vi "Find Center - Copy.vi"(7 "Tray Number":dbl format="%#_13g", 9 "XYZTheta":dbl[](array[numeric]), 11 "Gantry In":refnum<k24>) -> (1 "XYZTheta Centers":dbl[][](array[numeric]), 3 "Gantry Out":refnum<k24>)   [LabVIEW 2019, in "Assembly Tray.lvclass"]
uses:
  Assembly Tray.lvclass
  Find Tray.ctl
  Controller/Camera/Machine Vision.ctl
  C:/Program Files (x86)/Aerotech/A3200/LabVIEW/2010/Bin/Aerotech.A3200.dll
  Program Files (x86)/Aerotech/A3200/LabVIEW/2010/Bin/Aerotech.A3200.dll
  Controller/Camera/Camera.lvclass
  Controller/Motion/A3200/A3200.lvclass
panel:
  in  "BCG Values":T1={"Brightness"=128.0, "Contrast"=45.0, "Gamma"=1.0}
  in  "Machine Vision":T2=enum."Tray Fiducials"
  out "Right Fiducial":dbl[](array[numeric])
  out "Left Fiducial":dbl[](array[numeric])
  out "Gantry":dbl[](array[numeric])
  out "Sum":dbl[](array[numeric])
  out "Camera":dbl[](array[numeric])
  in  "Carrier Tray":T3
  out "Image":T4(plugin-control)
  out "Center":dbl[](array[numeric])
  in  "Position Number":i16
  in  "Go to Center":bool
  in  "Calculate":bool
  in  "Record Bottom":bool
  in  "Record Top":bool
  in  "Go to Bottom Fiducial":bool
  in  "Go to Top Fiducial":bool
  in  "Joystick":bool
  in  "Stop":bool
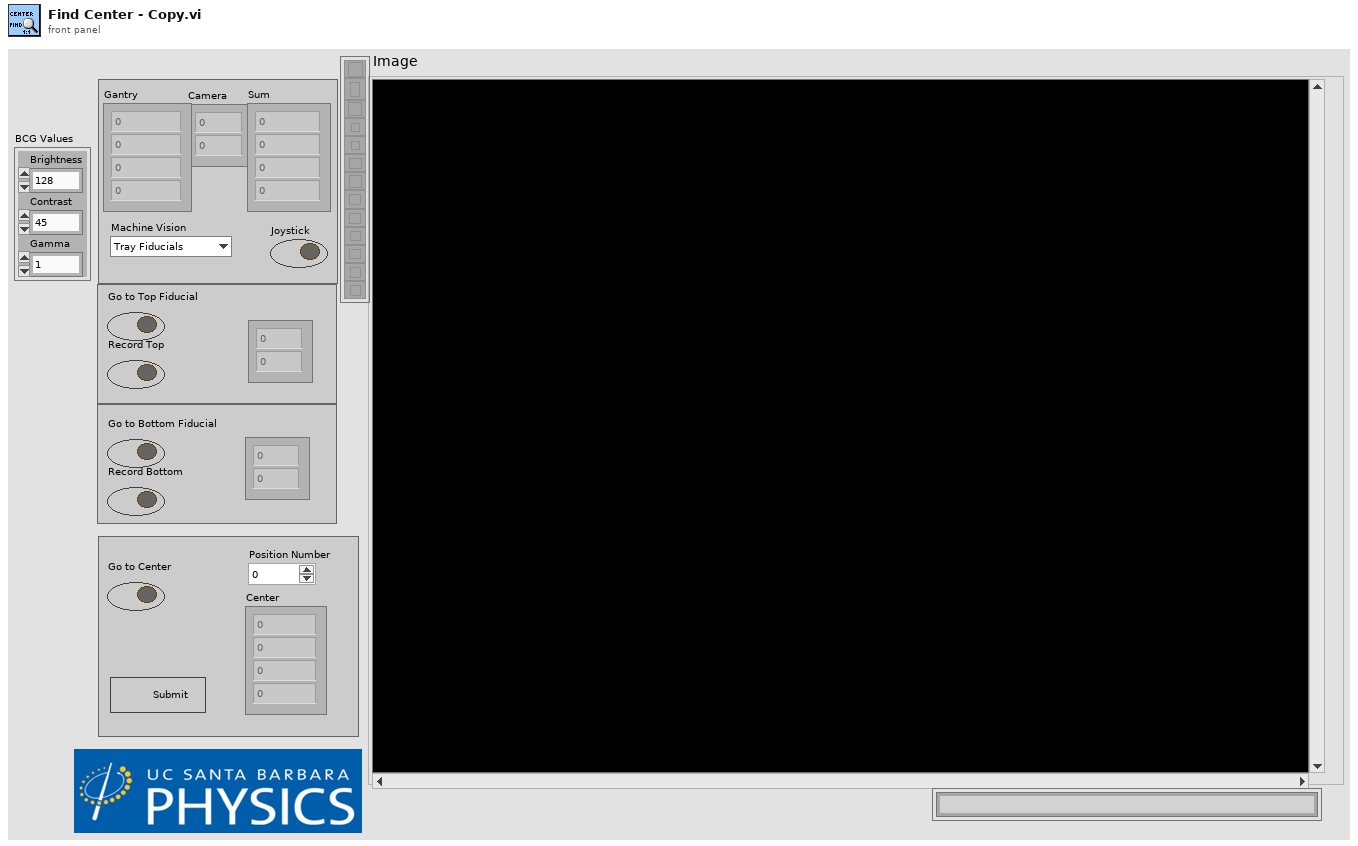
[diagram p1: front panel]
types:
  T1 = cluster{"Brightness":sgl, "Contrast":sgl, "Gamma":sgl}
  T2 = typedef "Camera.lvclass/Machine Vision.ctl" = enum16{"None", "Tray Fiducials", "HPK Silicon", "Hexaboard", "Corner (TL, BR)", "Corner (BL, TR)", "sensor TL", "sensor BL", "sensor TR", "sensor BR", "hexaboard TL", "hexaboard BL", "hexaboard TR", "hexaboard BR"}
  T3 = typedef "Assembly Tray.lvclass/Find Tray.ctl" = cluster{"Gantry Fiducials":dbl[], "Relative Coordinates":dbl[][], "Camera Fiducials":dbl[][], "XYZTheta Centers":dbl[][], "Workspace Center":dbl[], "Syringe Relative Coordinates":dbl[], "Gantry Region":dbl, "Fiducials Path":path, "New Fiducials":dbl[][], "Past Fiducials":dbl[][], "XYZTheta":dbl[], "Position":i32}
  T4 = typedef "IMAQ Image.ctl" = refnum<image>
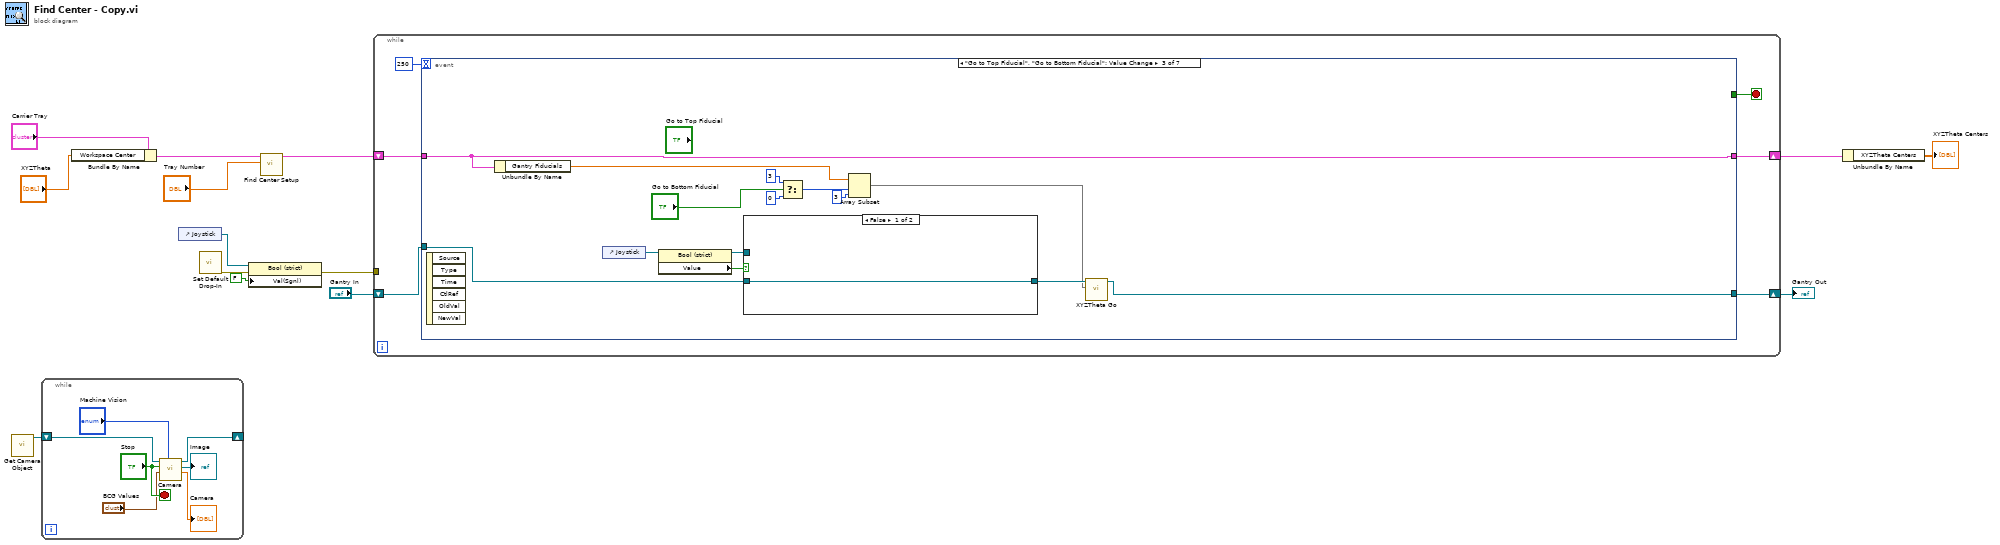
[diagram p0: block diagram]
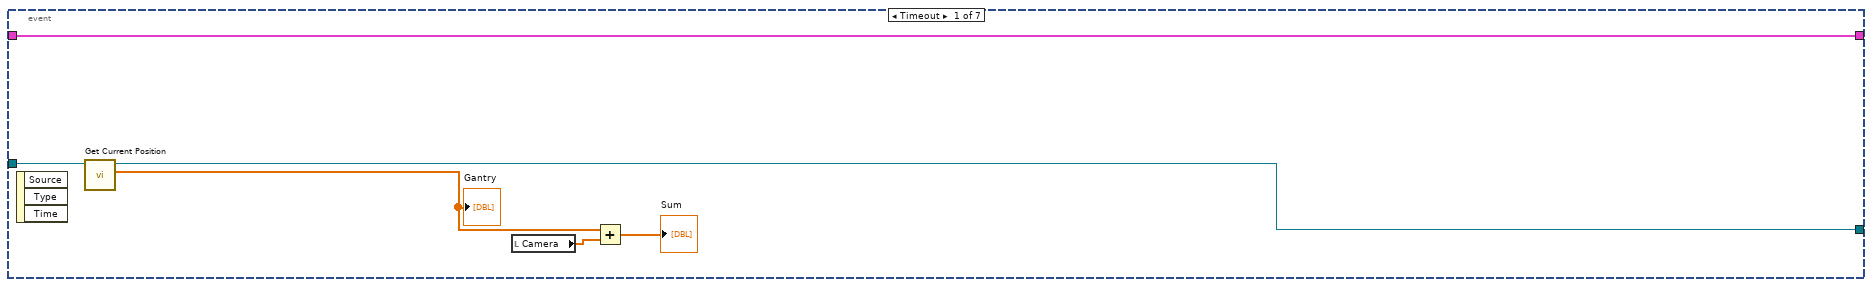
[diagram p2: hidden frame]
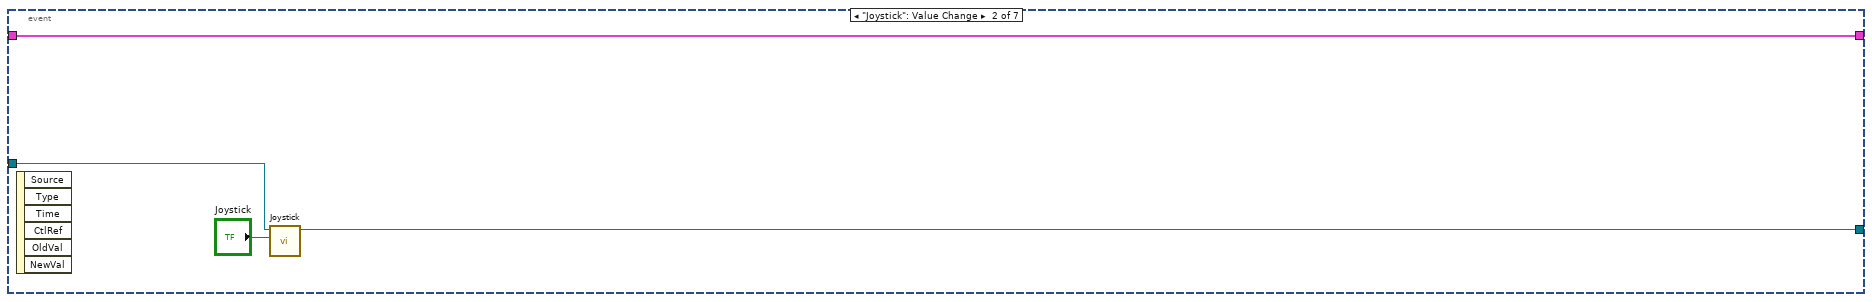
[diagram p3: hidden frame]
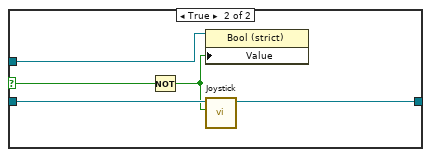
[diagram p4: hidden frame]
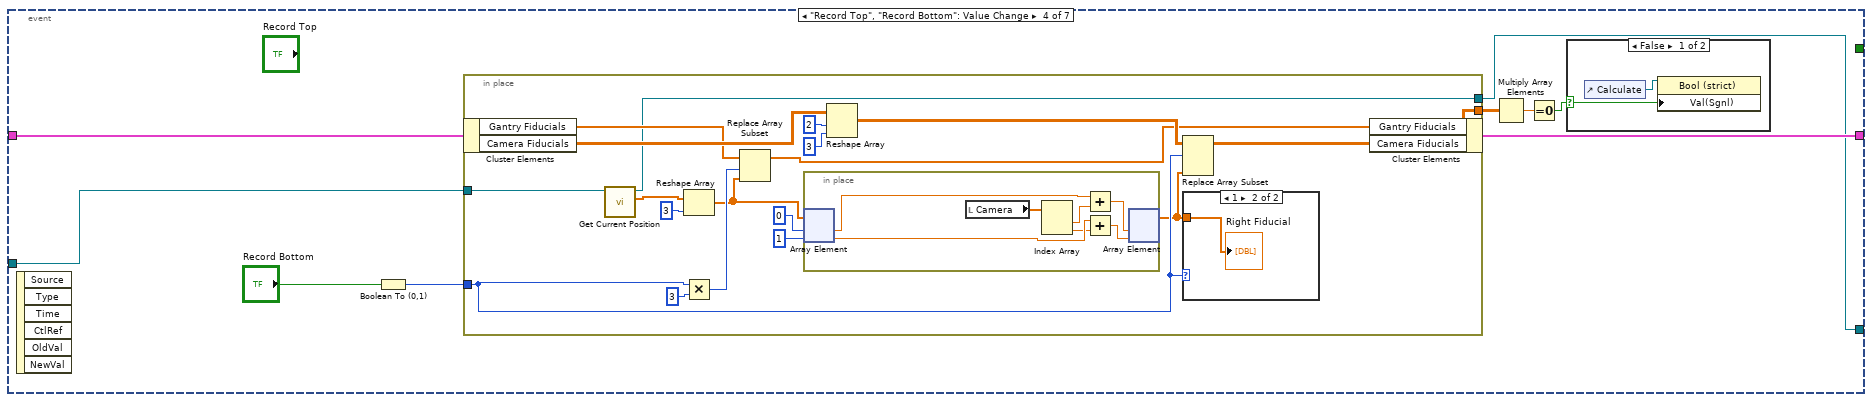
[diagram p5: hidden frame]
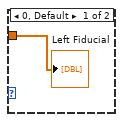
[diagram p7: hidden frame]
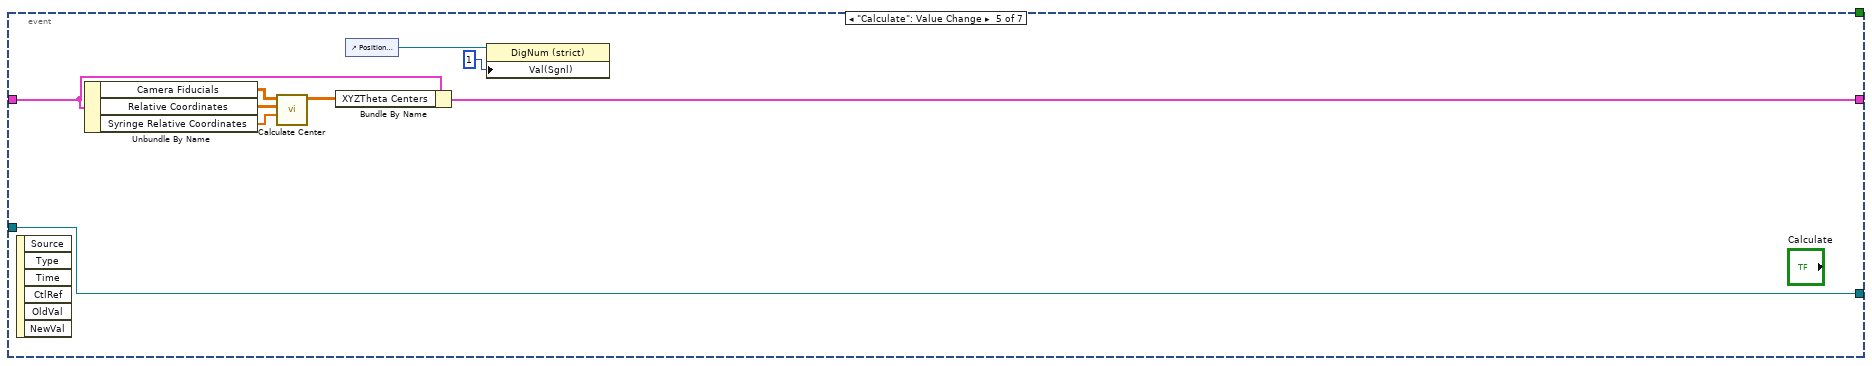
[diagram p8: hidden frame]
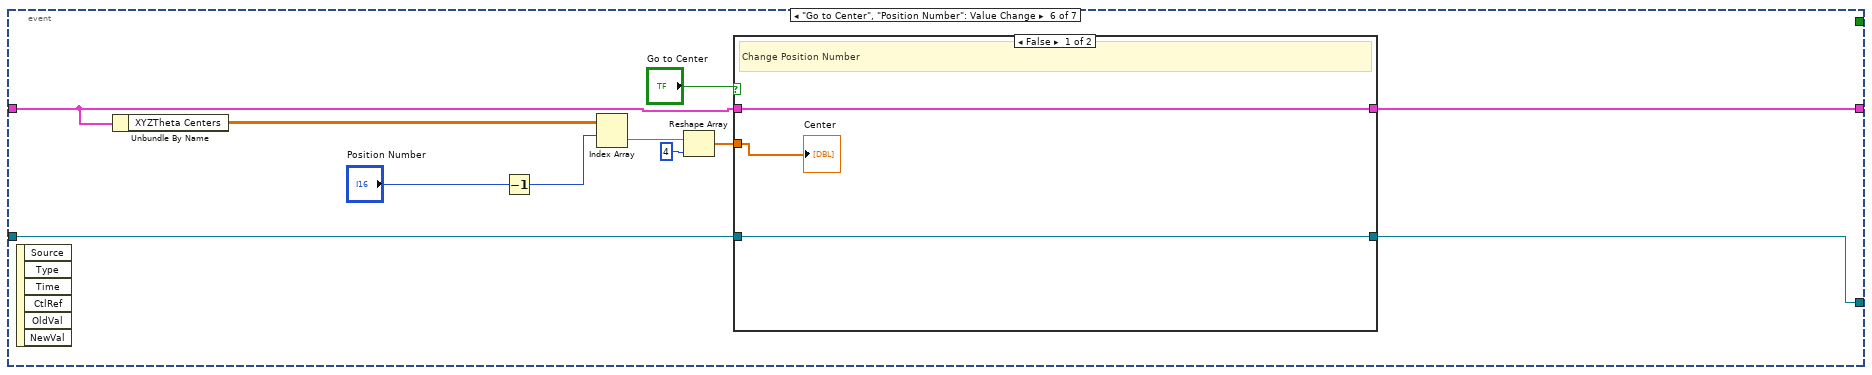
[diagram p9: hidden frame]
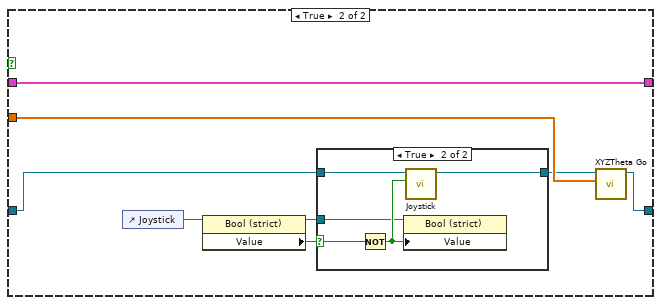
[diagram p10: hidden frame]
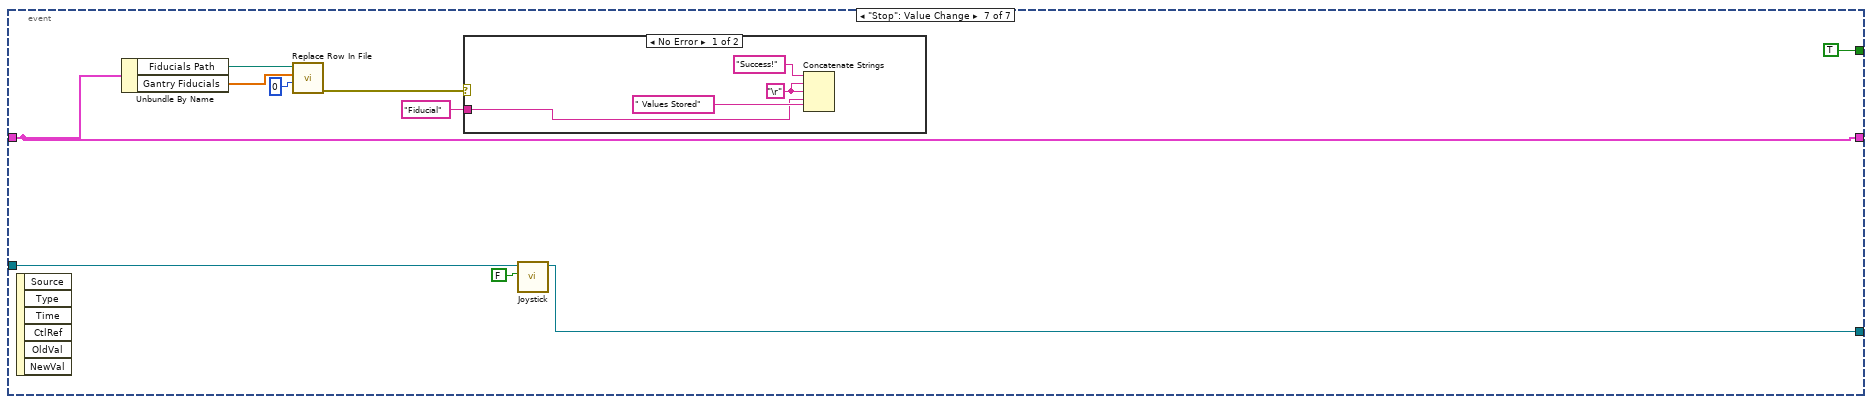
[diagram p12: hidden frame]
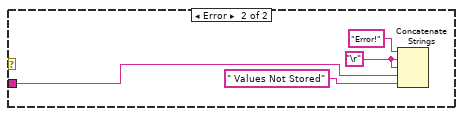
[diagram p13: hidden frame]
diagram:
  n1 = call "Get Camera Object.vi"() -> ("Camera out"=w3:refnum<class "Camera.lvclass">)  [unwired: 10 in, 1 out]
  n2 = while {
    shift-right: [w16] -> _
    shift-left: w3 -> [w21]
    stop <- "Stop" stop-if-true
    n3 = call "Camera.vi"("Machine Vision"="Machine Vision", "BCG Values"="BCG Values", "Stop"="Stop", "Camera in"=w21) -> ("Camera"=→"Camera":dbl[], "Image"=→"Image":T4, "Camera out"=w16:refnum<class "Camera.lvclass">)  [unwired: 4 in, 1 out]
  }
  n4 = Bundle By Name(cluster="Carrier Tray", "Workspace Center"="XYZTheta") -> (w8:T3)
  n5 = control-ref of="Joystick"() -> (w14:refnum<vi>)
  n6 = call "Set Default Drop-In.vi"() -> ("error out"=w6:errorcluster)  [unwired: 11 in]
  n7 = property class="Bool (strict)"(reference=w14, error in=w6, "Val(Sgnl)"=FALSE) -> (error out=w12:errorcluster)  [unwired: 1 out]
  n8 = call "Find Center Setup.vi"("Carrier Tray"=w8, "Tray Number"="Tray Number") -> ("Assembly Tray Out"=w11:T3)  [unwired: 8 in]
  n9 = while {
    shift-right: [w26] -> w10
    shift-left: w11 -> [w27]
    tunnel: w12 -> [_]
    shift-right: [w22] -> w1
    shift-left: "Gantry In" -> [w23]
    stop <- w25 stop-if-true
    n10 = event shown="[2] \"Go to Top Fiducial\", \"Go to Bottom Fiducial\": Value Change" {
      selector: _ -> [_ _ _ _ _ _ _]
      dyn-events: _ -> [_ _ _ _ _ _ _]
      timeout: 250 -> [_ _ _ _ _ _ _]
      tunnel: [w31 w37 w51 w66 w98 w111 w137] -> w26
      tunnel: w27 -> [w31 w37 w51 w60 w102 w112 w137]
      tunnel: [_ _ _ _ _ _ TRUE] -> w25
      tunnel: w23 -> [w30 w36 w43 w59 w96 w109 w138]
      tunnel: [w28 w34 w40 w58 w96 w105 w133] -> w22
      event Timeout {
        n11 = event-data() -> ()  [unwired: 1 in, 3 out]
        n12 = call "Get Current Position.vi"("Gantry In"=w30) -> ("XYZTheta Out"=w29:dbl[], "Gantry Out"=w28:refnum<k24>)  [unwired: 8 in, 1 out]
        "Gantry" <- w29
        n13 = local read "Camera"() -> (w33:dbl[])
        n14 = Add(x=w29, y=w33) -> (x+y=→"Sum":dbl[])
      }
      event "Joystick": Value Change {
        n15 = event-data() -> ()  [unwired: 1 in, 6 out]
        n16 = call "Joystick.vi"("Joystick"="Joystick", "Gantry In"=w36) -> ("Gantry Out"=w34:refnum<k24>)  [unwired: 8 in, 1 out]
      }
      event "Go to Top Fiducial", "Go to Bottom Fiducial": Value Change {
        n17 = event-data() -> ()  [unwired: 1 in, 6 out]
        n18 = Unbundle By Name(w51) -> ("Gantry Fiducials"=w39:dbl[])
        n19 = control-ref of="Joystick"() -> (w50:refnum<vi>)
        n20 = property class="Bool (strict)"(reference=w50) -> (reference out=w41:refnum<vi>, "Value"=w44:bool)  [unwired: 1 in, 1 out]
        n21 = case shown="False" w44 {
          selector: w44 -> [_ w57]
          tunnel: w43 -> [w52 w55]
          tunnel: [w52 w54] -> w42
          tunnel: w41 -> [_ w56]
          frame False {
          }
          frame True {
            n22 = Not(x=w57) -> (.not. x?=w53:bool)
            n23 = property class="Bool (strict)"(reference=w56, "Value"=w53) -> ()  [unwired: 1 in, 2 out]
            n24 = call "Joystick.vi"("Joystick"=w53, "Gantry In"=w55) -> ("Gantry Out"=w54:refnum<k24>)  [unwired: 8 in, 1 out]
          }
        }
        n25 = Select(t=3, s="Go to Bottom Fiducial", f=0) -> (s? t:f=w48:i32)
        n26 = Array Subset(array=w39, index=w48, length=3) -> (w38:dbl[])
        n27 = call "XYZTheta Go.vi"("XYZTheta In"=w38, "Gantry In"=w42) -> ("Gantry Out"=w40:refnum<k24>)  [unwired: 7 in, 2 out]
      }
      event "Record Top", "Record Bottom": Value Change {
        n28 = event-data() -> ()  [unwired: 1 in, 6 out]
        n29 = Boolean To (0,1)(Boolean="Record Bottom") -> (0, 1=w62:i16)
        n30 = in-place {
          in-place-border: [w80] -> w63
          in-place-border: w62 -> [w73]
          in-place-border: w59 -> [w75]
          in-place-border: [w74] -> w58
          n31 = in-place-cluster #1(w60) -> ("Gantry Fiducials"=w77:dbl[], "Camera Fiducials"=w84:dbl[][])
          n32 = call "Get Current Position.vi"("Gantry In"=w75) -> ("XYZTheta Out"=w78:dbl[], "Gantry Out"=w74:refnum<k24>)  [unwired: 8 in, 1 out]
          n33 = Reshape Array(w78, 3 ("dimension size")) -> (w70:dbl[])
          n34 = Multiply(x=w73, y=i16 3) -> (x*y=w71:i16)
          n35 = Replace Array Subset(array=w77, new element=w70, index=w71) -> (w76:dbl[])
          n36 = in-place {
            n37 = in-place-array #2(w70, 0, 1) -> (w92:dbl, w90:dbl)
            n38 = local read "Camera"() -> (w93:dbl[])
            n39 = Index Array(array=w93) -> (element #1=w91:dbl, element #2=w89:dbl)  [unwired: 2 in]
            n40 = Add(x=w92, y=w91) -> (x+y=w87:dbl)
            n41 = Add(x=w90, y=w89) -> (x+y=w88:dbl)
            n42 = in-place-array #2(w87, w88) -> (w69:dbl[])  [unwired: 2 out]
          }
          n43 = Reshape Array(w84, 2 ("length"), 3 ("dimension size")) -> (w83:dbl[][])
          n44 = Replace Array Subset(array=w83, new element=w69, index (row)=w73) -> (w80:dbl[][])  [unwired: 1 in]
          n45 = case shown="1" w73 {
            tunnel: w69 -> [w94 w95]
            frame 0, Default {
              "Left Fiducial" <- w94
            }
            frame 1 {
              "Right Fiducial" <- w95
            }
          }
          n46 = in-place-cluster #1("Gantry Fiducials"=w76, "Camera Fiducials"=w80) -> (w66:T3)
        }
        n47 = Multiply Array Elements(1:w63) -> (0:w65:dbl)
        n48 = Equal To 0?(x=w65) -> (x = 0?=w64:bool)
        n49 = case shown="False" w64 {
          selector: w64 -> [w67 _]
          frame False {
            n50 = control-ref of="Calculate"() -> (w68:refnum<vi>)
            n51 = property class="Bool (strict)"(reference=w68, "Val(Sgnl)"=w67) -> ()  [unwired: 1 in, 2 out]
          }
          frame True {
          }
        }
      }
      event "Calculate": Value Change {
        n52 = event-data() -> ()  [unwired: 1 in, 6 out]
        n53 = Unbundle By Name(w102) -> ("Camera Fiducials"=w101:dbl[][], "Relative Coordinates"=w100:dbl[][], "Syringe Relative Coordinates"=w97:dbl[])
        n54 = call "Calculate Center.vi"("Syringe Coordinates"=w97, "Relative Coordinates"=w100, "Fiducial Measurements"=w101) -> ("XYZTheta Centers"=w99:dbl[][])  [unwired: 8 in]
        n55 = Bundle By Name(cluster=w102, "XYZTheta Centers"=w99) -> (w98:T3)
        n56 = control-ref of="Position Number"() -> (w104:refnum<vi>)
        n57 = property class="DigNum (strict)"(reference=w104, "Val(Sgnl)"=i16 1 ("Value (Signaling)")) -> ()  [unwired: 1 in, 2 out]
      }
      event "Go to Center", "Position Number": Value Change {
        n58 = event-data() -> ()  [unwired: 1 in, 6 out]
        n59 = Unbundle By Name(w112) -> ("XYZTheta Centers"=w115:dbl[][])
        n60 = Decrement(x="Position Number") -> (x-1=w113:i16)
        n61 = Index Array(array=w115, index (row)=w113) -> (element=w107:dbl[])  [unwired: 1 in]
        n62 = Reshape Array(w107, u32 4) -> (w106:dbl[])
        n63 = case shown="False" "Go to Center" {
          tunnel: w106 -> [w118 w124]
          tunnel: w112 -> [w117 w126]
          tunnel: [w117 w126] -> w111
          tunnel: w109 -> [w116 w120]
          tunnel: [w116 w125] -> w105
          frame False {
            # "Change Position Number"
            "Center" <- w118
          }
          frame True {
            n64 = control-ref of="Joystick"() -> (w123:refnum<vi>)
            n65 = property class="Bool (strict)"(reference=w123) -> (reference out=w121:refnum<vi>, "Value"=w122:bool)  [unwired: 1 in, 1 out]
            n66 = case shown="True" w122 {
              selector: w122 -> [_ w132]
              tunnel: w120 -> [w127 w131]
              tunnel: [w127 w130] -> w119
              tunnel: w121 -> [_ w128]
              frame False {
              }
              frame True {
                n67 = Not(x=w132) -> (.not. x?=w129:bool)
                n68 = property class="Bool (strict)"(reference=w128, "Value"=w129) -> ()  [unwired: 1 in, 2 out]
                n69 = call "Joystick.vi"("Joystick"=w129, "Gantry In"=w131) -> ("Gantry Out"=w130:refnum<k24>)  [unwired: 8 in, 1 out]
              }
            }
            n70 = call "XYZTheta Go.vi"("XYZTheta In"=w124, "Gantry In"=w119) -> ("Gantry Out"=w125:refnum<k24>)  [unwired: 7 in, 2 out]
          }
        }
      }
      event "Stop": Value Change {
        n71 = event-data() -> ()  [unwired: 1 in, 6 out]
        n72 = Unbundle By Name(w137) -> ("Fiducials Path"=w135:path, "Gantry Fiducials"=w136:dbl[])
        n73 = call "Replace Row In File.vi"("Index"=0, "Insert Array"=w136, "Path"=w135) -> ("error out"=w141:errorcluster)  [unwired: 8 in]
        n74 = case shown="No Error" w141 {
          tunnel: "Fiducial" -> [w143 w150]
          frame No Error {
            w144 = "\r"
            n75 = Concatenate Strings("Success!", w144, w144, w143, " Values Stored") -> ()  [unwired: 1 out]
          }
          frame Error {
            w147 = "\r"
            n76 = Concatenate Strings("Error!", w147, w147, w150, " Values Not Stored") -> ()  [unwired: 1 out]
          }
        }
        n77 = call "Joystick.vi"("Joystick"=FALSE, "Gantry In"=w138) -> ("Gantry Out"=w133:refnum<k24>)  [unwired: 8 in, 1 out]
      }
    }
  }
  "Gantry Out" <- w1
  n78 = Unbundle By Name(w10) -> ("XYZTheta Centers"=→"XYZTheta Centers":dbl[][])
